vi "sample9(DXL).vi"() -> ()   [LabVIEW 2020]
panel:
  in  "OffsetTime":u32=500
  in  "Baudrate":u32=57600 min=9600 max=12000000
  in  "COM":refnum<visa-resource-name> caption="COMポート"
  out "ids":u8[](array[numeric])
  in  "angle":dbl(knob) scale=-180.0..180.0
  in  "停止":bool
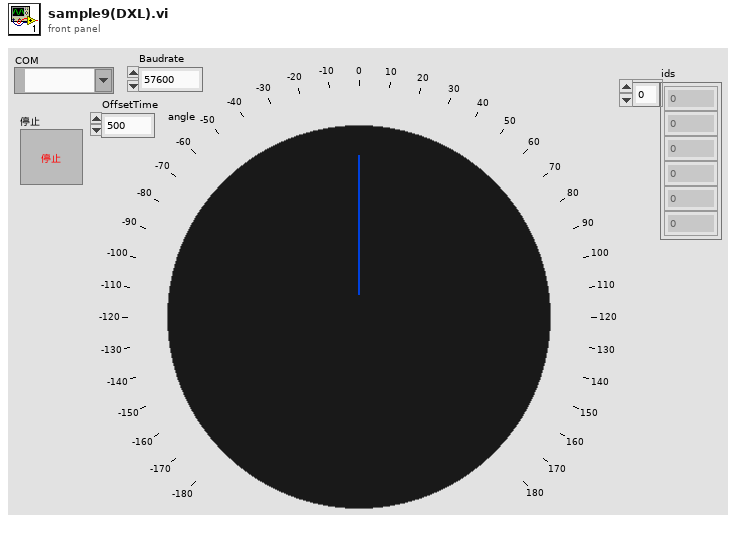
[diagram p1: front panel]
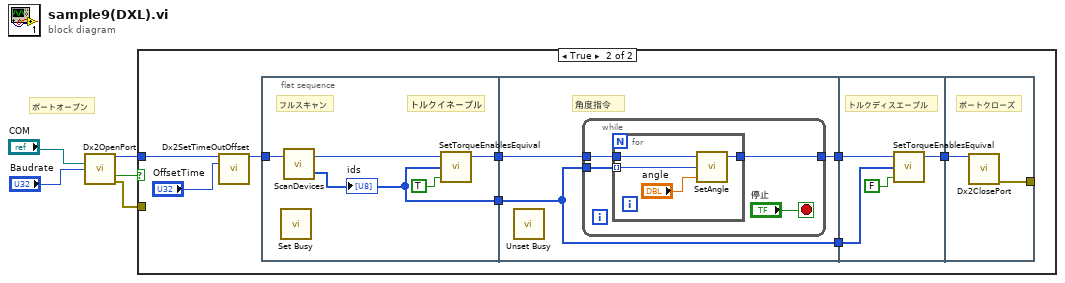
[diagram p0: block diagram]
diagram:
  # "ポートオープン"
  n1 = call "Dx2OpenPort.vi"("port"="COM", "baudrate"="Baudrate") -> ("dvid"=w4:u32, "成功"=w5:bool, "エラー出力"=w3:errorcluster)  [unwired: 11 in]
  n2 = case shown="TRUE" w5 {
    tunnel: w4 -> [_ w8]
    tunnel: w3 -> [_ _]
    frame False {
    }
    frame True {
      n3 = call "Dx2SetTimeOutOffset.vi"("dvid in"=w8, "OffsetTime"="OffsetTime") -> ("dvid out"=w7:u32)  [unwired: 12 in, 1 out]
      n4 = flat-sequence {
        tunnel: [w15] -> w13
        tunnel: w7 -> [w18]
        tunnel: [w14] -> w12
        tunnel: w13 -> [w21]
        tunnel: [w20] -> w11
        tunnel: w12 -> [w19]
        tunnel: [w19] -> w9
        tunnel: w11 -> [w31]
        tunnel: [w32] -> w10
        tunnel: w9 -> [w30]
        tunnel: [w34] -> _
        tunnel: w10 -> [w35]
        frame #0 {
          # "トルクイネーブル"
          # "フルスキャン"
          n5 = call <vilib>:"Set Busy.vi"() -> ()  [unwired: 10 in, 2 out]
          n6 = call "ScanDevices.vi"("dvid in"=w18) -> ("ids"=w14:u8[], "dvid out"=w17:u32)  [unwired: 1 in]
          "ids" <- w14
          n7 = call "SetTorqueEnablesEquival.vi"("torqueenable"=TRUE, "ids"=w14, "dvid in"=w17) -> ("dvid out"=w15:u32)  [unwired: 1 in, 1 out]
        }
        frame #1 {
          # "角度指令"
          n8 = call <vilib>:"Unset Busy.vi"() -> ()  [unwired: 11 in, 1 out]
          n9 = while {
            tunnel: w21 -> [w25]
            tunnel: [w23] -> w20
            tunnel: w19 -> [w22]
            stop <- "停止" stop-if-true
            n10 = for {
              tunnel: w25 -> [w29]
              tunnel: [w27] -> w23
              tunnel: w22 -> [w26] mode=indexing
              n11 = call "SetAngle.vi"("angle"="angle", "Target ID"=w26, "dvid in"=w29) -> ("dvid out"=w27:u32)  [unwired: 1 in, 1 out]
            }
          }
        }
        frame #2 {
          # "トルクディスエーブル"
          n12 = call "SetTorqueEnablesEquival.vi"("torqueenable"=FALSE, "ids"=w30, "dvid in"=w31) -> ("dvid out"=w32:u32)  [unwired: 1 in, 1 out]
        }
        frame #3 {
          # "ポートクローズ"
          n13 = call "Dx2ClosePort.vi"("dvid"=w35) -> ("エラー出力"=w34:errorcluster)  [unwired: 13 in, 1 out]
        }
      }
    }
  }
